vi "EthernetWriterTest.vi"() -> ()   [LabVIEW 2025]
uses:
  <vilib>/xnet/xnet.llb/XNET Frame Type Ethernet.ctl
  <vilib>/xnet/xnet.llb/XNET Create Session (Frame Output Stream).vi
  <vilib>/xnet/xnet.llb/XNET Write (Frame Ethernet).vi
  Automotive Ethernet Bus Monitor/Automotive Ethernet Bus Monitor.lvclass
panel:
  in  "Ethertype 4":u16=3 format="%.0x"
  in  "Ethertype 3":u16=2 format="%.0x"
  in  "payload 4":string="medium payload"
  in  "payload 3":string="payload1"
  in  "Stop 2":bool
  in  "payload 2":string="payload2 is so much longer than payload1"
  in  "destination MAC address 2":cluster{u8, u8, u8, u8, u8, u8}={255, 255, 255, 255, 255, 255} {"?" format="%.0x"; "?" format="%.0x"; "?" format="%.0x"; "?" format="%.0x"; "?" format="%.0x"; "?" format="%.0x"}
  in  "Has VLAN Tag 2":bool=TRUE
  in  "Ethertype 2":u16=1 format="%.0x"
  in  "VID 2":u16=2
  in  "priority 2":u8=3
  in  "loop 2":bool
  out "Number of Frames Sent 2":u32
  in  "Write Frame 2":bool
  in  "Interface":refnum<k21>="ENET1"
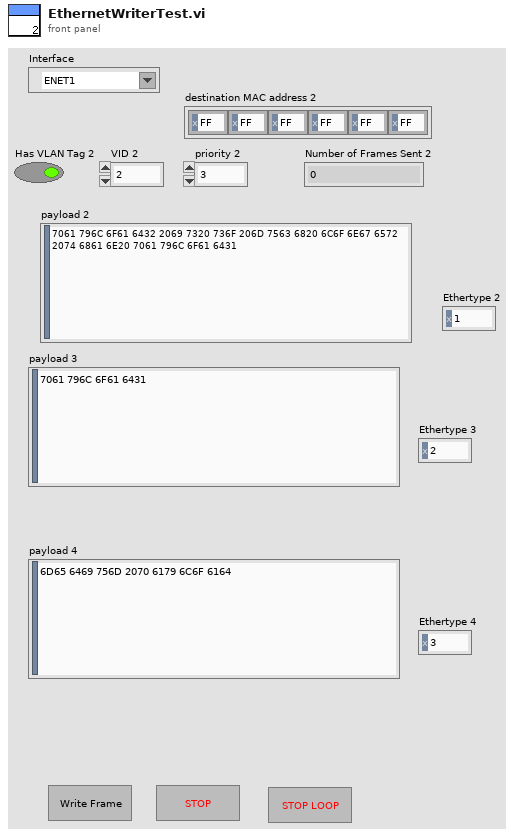
[diagram p1: front panel]
types:
  T1 = typedef "XNET Frame Type Ethernet.ctl" = u16
  T2 = cluster{"local timestamp":timestamp, "network timestamp":timestamp, "frame data":u8[], "fcs":u32, "type":T1, "network synced?":bool, "receive?":bool, "transmit?":bool, "error?":bool}
  T3 = cluster{"destination MAC address":cluster{u8, u8, u8, u8, u8, u8}, "source MAC address":cluster{u8, u8, u8, u8, u8, u8}, "Has VLAN Tag":bool, "VLAN Tag":cluster{"TPID":u16, "priority":u8, "DEI":bool, "VID":u16}, "Ethertype":u16}
  T4 = cluster{"TPID":u16, "priority":u8, "DEI":bool, "VID":u16}
  T5 = cluster{"local timestamp":timestamp, "network timestamp":timestamp, "frame data":u8[], "fcs":u32, "type":T1, "network synced?":bool, "receive?":bool, "transmit?":bool, "error?":bool}[]
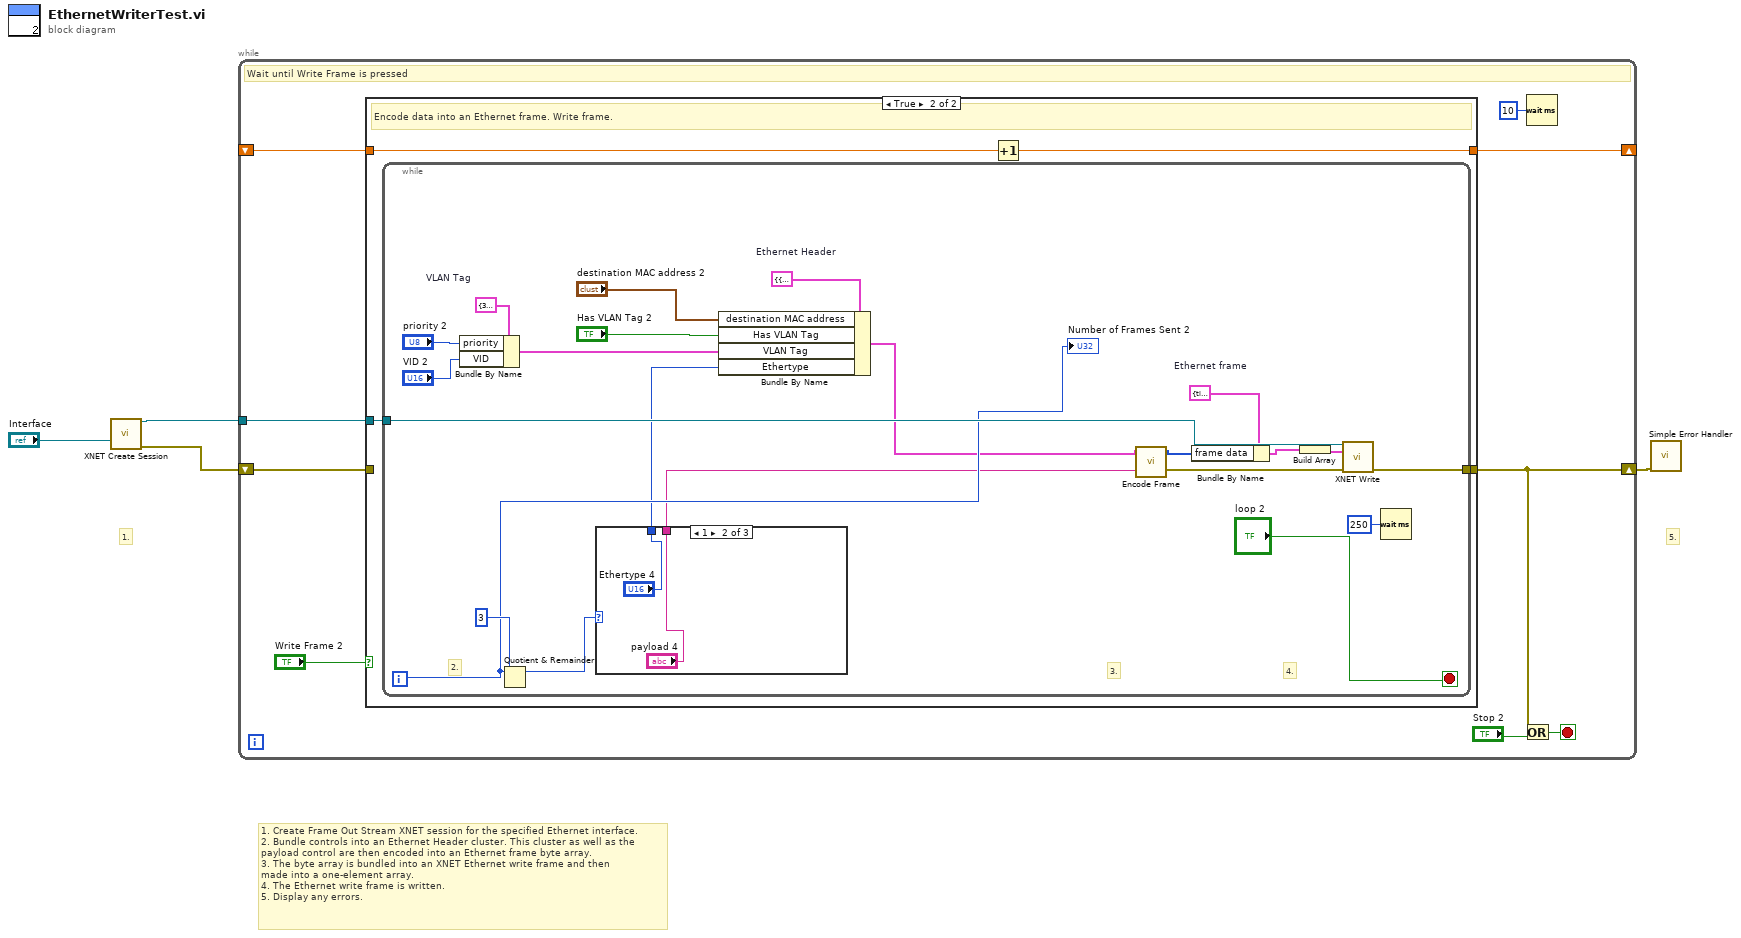
[diagram p0: block diagram]
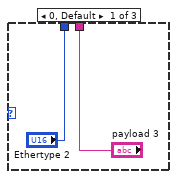
[diagram p3: hidden frame]
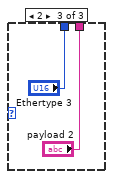
[diagram p4: hidden frame]
diagram:
  # "1. Create Frame Out Stream XNET session for the specified Ethernet interface.\n2. Bundle controls into an Ethernet Header cluster. This cluster as well as the\npayload control are then encoded into an Ethernet frame byte array.\n3. The byte array is bundled into an XNET Ethernet write frame and then\nmade into a one-element array.\n4. The Ethernet write frame is written.\n5. Display any errors."
  # "5."
  # "1."
  n1 = call-poly <vilib>:"XNET Create Session.vi"("interface"="Interface") -> ("session out"=w3:refnum<k21>, "error out"=w2:errorcluster)  [unwired: 13 in]
  n2 = while {
    shift-right: [w9] -> w1
    shift-left: w2 -> [w11]
    tunnel: w3 -> [w12]
    shift-right: [w5] -> _
    shift-left: _ -> [w6]
    stop <- w8 stop-if-true
    # "Wait until Write Frame is pressed"
    n3 = case shown="True" "Write Frame 2" {
      tunnel: w12 -> [_ w19]
      tunnel: w11 -> [w15 _]
      tunnel: [w15 w18] -> w9
      tunnel: w6 -> [w14 w17]
      tunnel: [w14 w16] -> w5
      frame False {
      }
      frame True {
        # "Encode data into an Ethernet frame. Write frame."
        n4 = while {
          tunnel: w19 -> [w41]
          tunnel: [w38] -> w18
          i -> [w25]
          stop <- "loop 2" stop-if-true
          w32 = T2 {"local timestamp"=timestamp(0 s since 1904-01-01), "network timestamp"=timestamp(0 s since 1904-01-01), "frame data"=[], "fcs"=0, "type"=0, "network synced?"=FALSE, "receive?"=FALSE, "transmit?"=FALSE, "error?"=FALSE}  # Ethernet frame
          w37 = T3 {"destination MAC address"={0, 0, 0, 0, 0, 0}, "source MAC address"={0, 0, 0, 0, 0, 0}, "Has VLAN Tag"=FALSE, "VLAN Tag"={"TPID"=33024, "priority"=0, "DEI"=FALSE, "VID"=0}, "Ethertype"=0}  # Ethernet Header
          w36 = T4 {"TPID"=33024, "priority"=0, "DEI"=FALSE, "VID"=0}  # VLAN Tag
          # "4."
          # "3."
          # "2."
          n5 = Bundle By Name(cluster=w36, "priority"="priority 2", "VID"="VID 2") -> (w35:T4)
          n6 = Quotient & Remainder(x=w25, y=3) -> (x-y*floor(x/y)=w27:i32)  [unwired: 1 out]
          n7 = case shown="1" w27 {
            tunnel: ["payload 3" "payload 4" "payload 2"] -> w21
            tunnel: ["Ethertype 2" "Ethertype 4" "Ethertype 3"] -> w24
            frame 0, Default {
            }
            frame 1 {
            }
            frame 2 {
            }
          }
          n8 = Bundle By Name(cluster=w37, "destination MAC address"="destination MAC address 2", "Has VLAN Tag"="Has VLAN Tag 2", "VLAN Tag"=w35, "Ethertype"=w24) -> (w23:T3)
          n9 = call "Encode Frame.vi"("payload"=w21, "Ethernet Header"=w23) -> ("error out"=w20:errorcluster, "frame data"=w22:u8[])  [unwired: 8 in]
          n10 = Bundle By Name(cluster=w32, "frame data"=w22) -> (w31:T2)
          n11 = Build Array(w31) -> (w30:T5)
          n12 = call-poly <vilib>:"XNET Write.vi"("session in"=w41, "data"=w30, "error in (no error)"=w20) -> ("error out"=w38:errorcluster)  [unwired: 11 in, 1 out]
          n13 = Wait (ms)(milliseconds to wait=u32 250) -> ()  [unwired: 1 out]
          "Number of Frames Sent 2" <- w25
        }
        n14 = Increment(x=w17) -> (x+1=w16:dbl)
      }
    }
    n15 = Or(x=w9, y="Stop 2") -> (x .or. y?=w8:bool)
    n16 = Wait (ms)(milliseconds to wait=u32 10) -> ()  [unwired: 1 out]
  }
  n17 = call <vilib>:"Simple Error Handler.vi"("error in (no error)"=w1) -> ()  [unwired: 4 in, 5 out]
